vi "pH电极校准.vi"() -> ()   [LabVIEW 2016, in "斯坦道多参数.lvlib"]
uses:
  <vilib>/Utility/miscctls.llb/LVPointTypeDef.ctl
  <vilib>/Analysis/NI_AALBase.lvlib
panel:
  out "通讯状态":string
  in  "电极状态标志":u16(ring) items=["OK", "第一点校正通过", "第二点校正通过", "校正失败,电极零点超出范围", "校正失败,电极斜率超出范围", "第三点校正通过"]
  in  "三点标液3":u16(ring)=6 caption="标液3" items=["TECH4.00", "TECH7.00", "TECH10.00", "NIST1.68", "NIST4.01", "NIST6.86", "NIST9.18", "NIST12.68"]
  in  "三点标液2":u16(ring)=5 caption="标液2" items=["TECH4.00", "TECH7.00", "TECH10.00", "NIST1.68", "NIST4.01", "NIST6.86", "NIST9.18", "NIST12.68"]
  in  "三点标液1":u16(ring)=4 caption="标液1" items=["TECH4.00", "TECH7.00", "TECH10.00", "NIST1.68", "NIST4.01", "NIST6.86", "NIST9.18", "NIST12.68"]
  out "第三点校准值":dbl
  in  "校准停止":bool
  in  "校准启动":bool
  out "第二点校准值":dbl
  out "第一点校准值":dbl
  out "提示":string
  in  "校准模式":enum16{"两点校准", "单点校准", "三点校准"}(ring)
  out "最小值":sgl format="%#.2f"
  out "最大值":sgl format="%#.2f"
  out "变异系数":dbl format="%#.6f"
  out "standard deviation":dbl caption="标准差" format="%#.2f"
  out "mean":dbl caption="均值" format="%#.2f"
  out "波形图表":sgl(graph) caption="历史曲线"
  out "当前检测值":dbl format="%#.2g"
  out "标液2":dbl
  out "标液1":dbl
  out "当前信号值":dbl format="%#.2g"
  out "偏移值补偿":dbl format="%#.2g"
  out "电极斜率":dbl
  out "电极零点":dbl
  # "酸碱度电极设定"
  # "mV"
  # "mV"
  # "%"
  # "pH"
  # "请选择校准模式:"
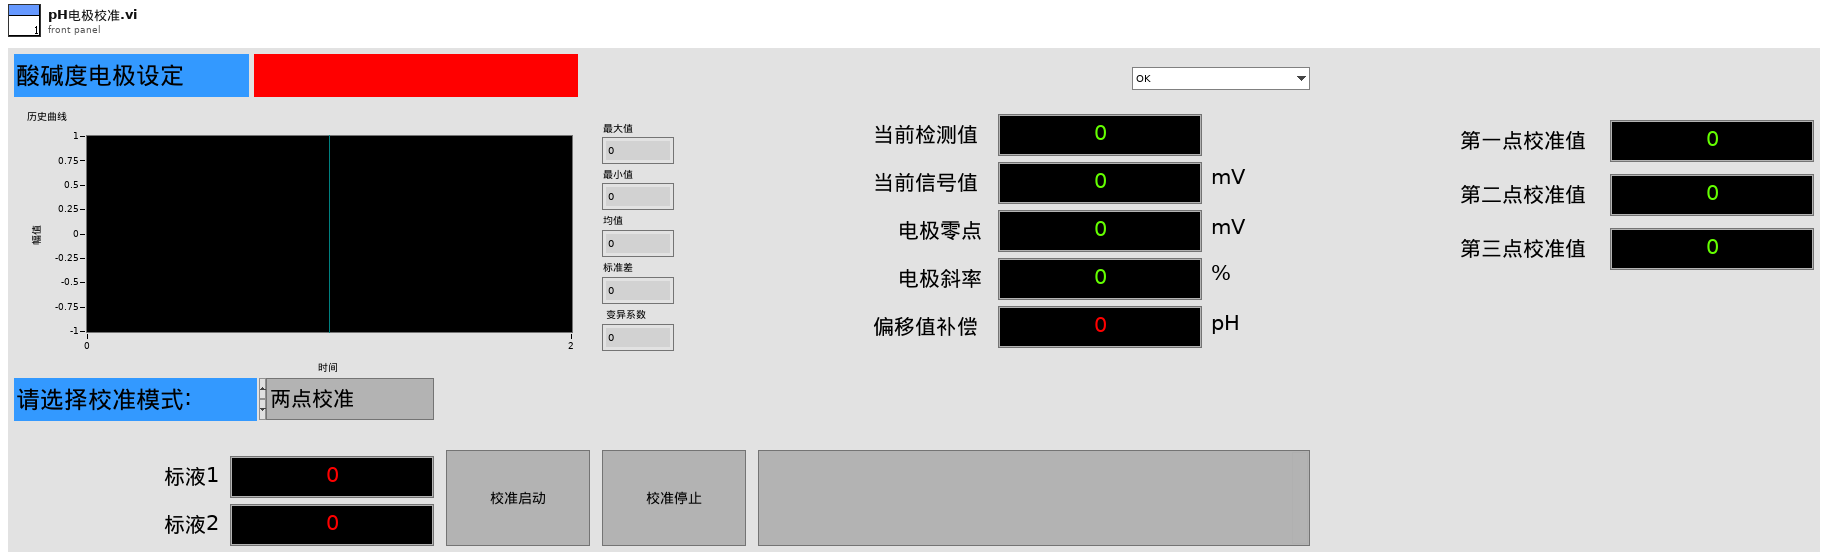
[diagram p1: front panel]
types:
  T1 = typedef "LVPointTypeDef.ctl" = cluster{"Horizontal":i16, "Vertical":i16}
  T2 = typedef "斯坦道多参数.lvlib/校准步骤.ctl" = enum16{"待机", "放置第一点标液", "第一点校准启动", "第一点校准写入", "第一点校准失败", "放置第二点标液", "第二点校准启动", "第二点校准写入", "第二点校准失败", "放置第三点标液", "第三点校准启动", "第三点校准写入", "第三点校准失败", "校准结果写入", "校准结束"}
  T3 = cluster{"电极状态标志":u16, "电极型号标志":u16, "酸碱度测量值":sgl, "温度测量值":sgl, "酸碱度信号值":sgl, "温度信号值":sgl, "酸碱度偏移修正值":sgl, "温度偏移修正值":sgl, "手动温度补偿值":sgl, "酸碱度电极零点":sgl, "酸碱度电极斜率":sgl, "第1点标准值记录":sgl, "第1点信号值记录":sgl, "第1点温度值记录":sgl, "第2点标准值记录":sgl, "第2点信号值记录":sgl, "第2点温度值记录":sgl, "命令滤波设定":u16, "温度模式":enum16{"ATC", "MTC"}, "生产批次":u16, "电极序号":u16, "串口地址":u16, "串口波特率":enum16{"9600", "19200", "115200"}, "串口校验位":enum16{"NONE", "ODD", "EVEN"}, "串口停止位":enum16{"1bit", "2bit"}, "第一点标准值":sgl, "第二点标准值":sgl}
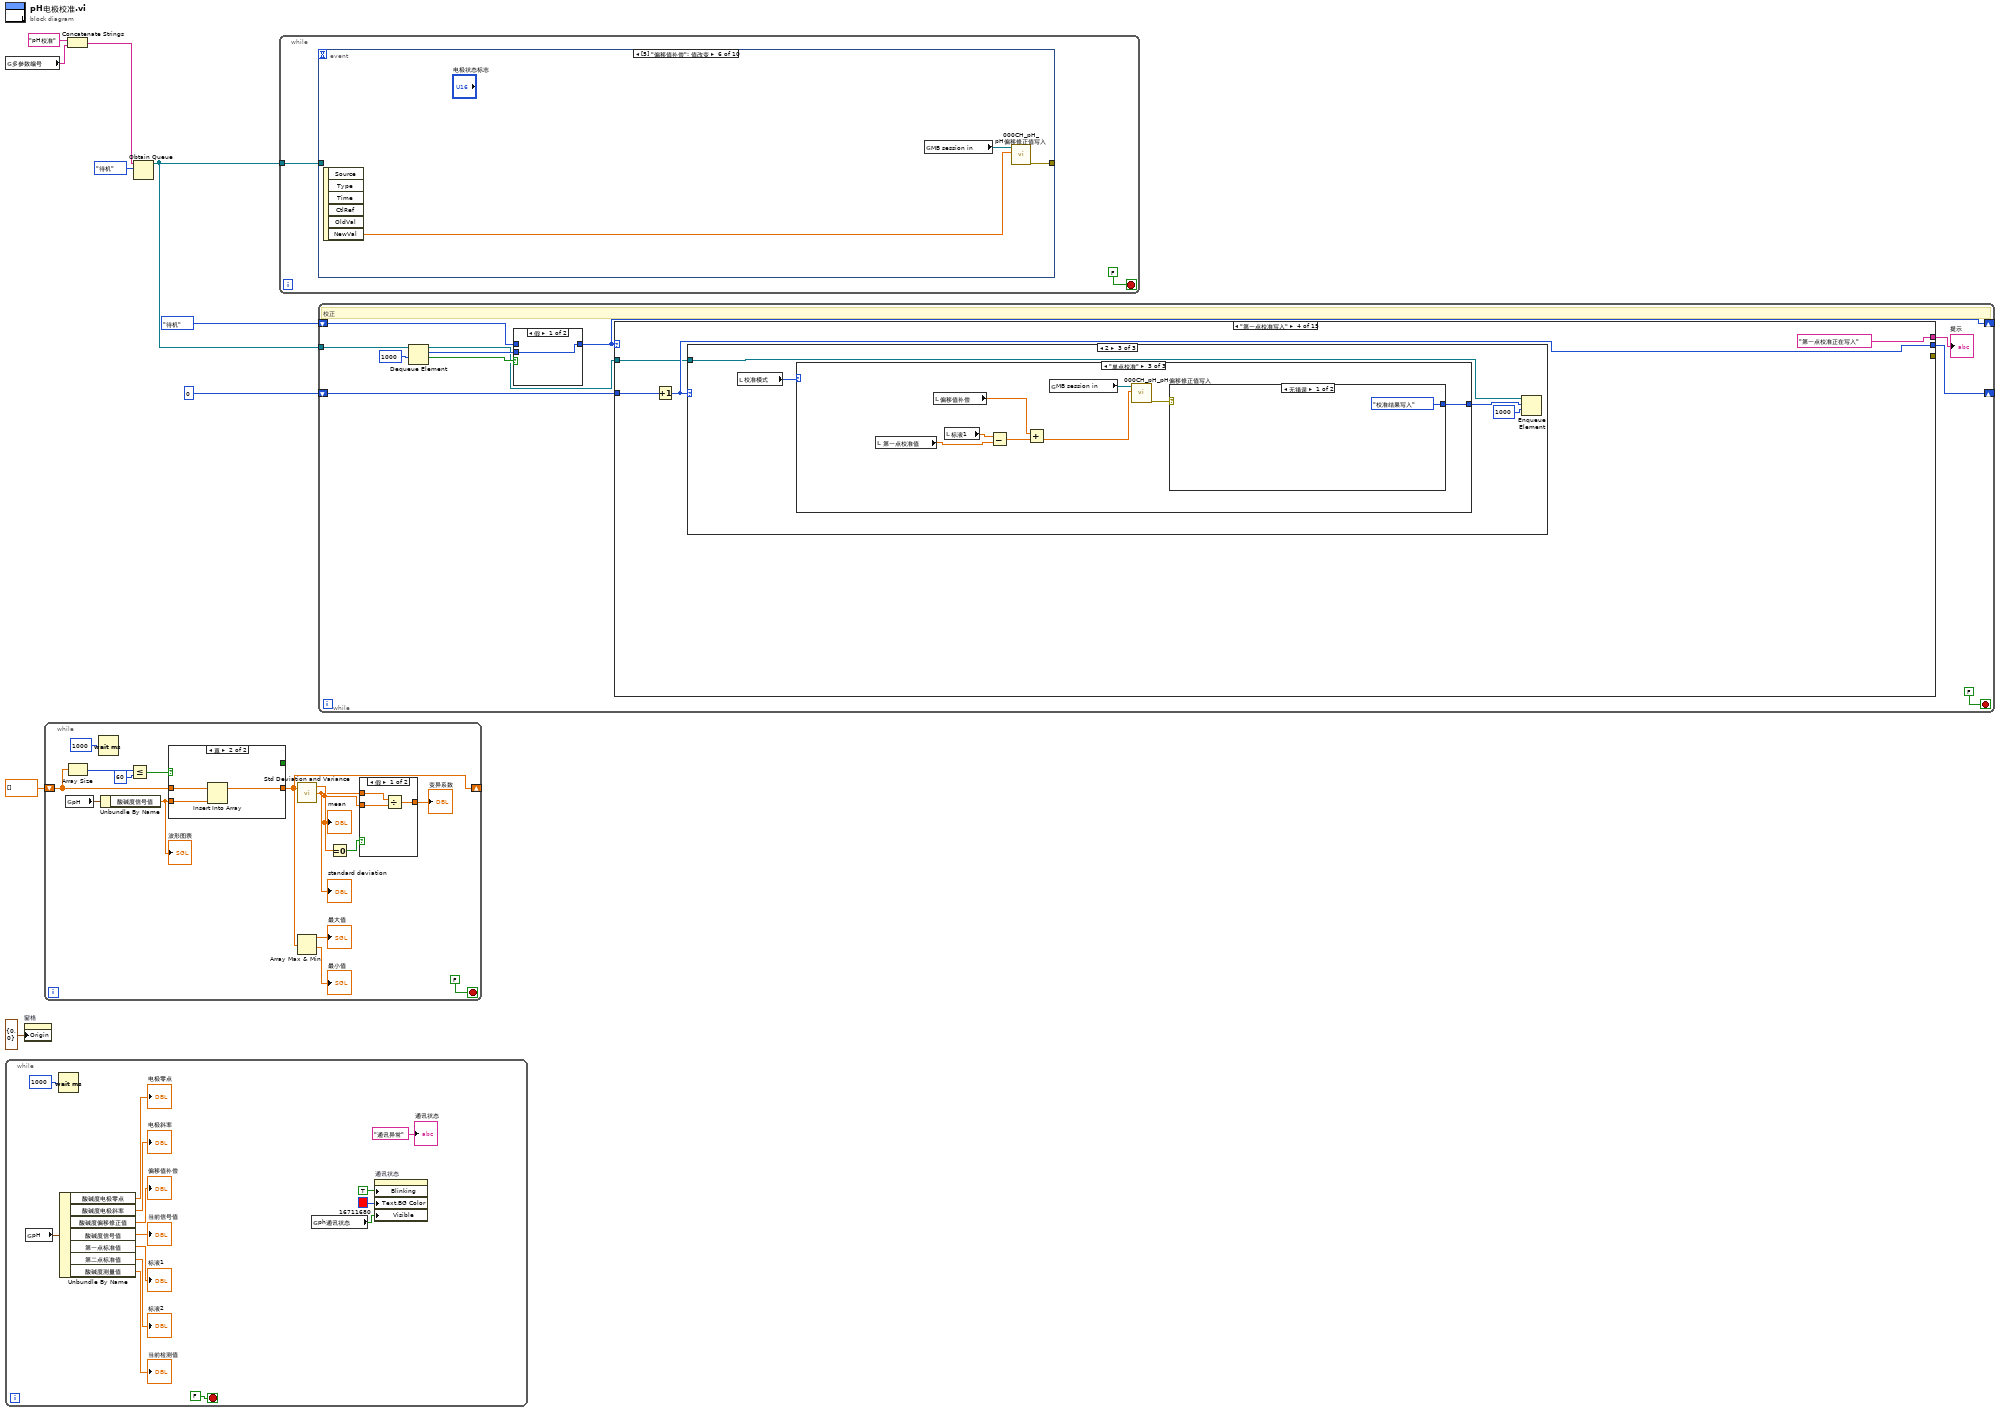
[diagram p0: block diagram]
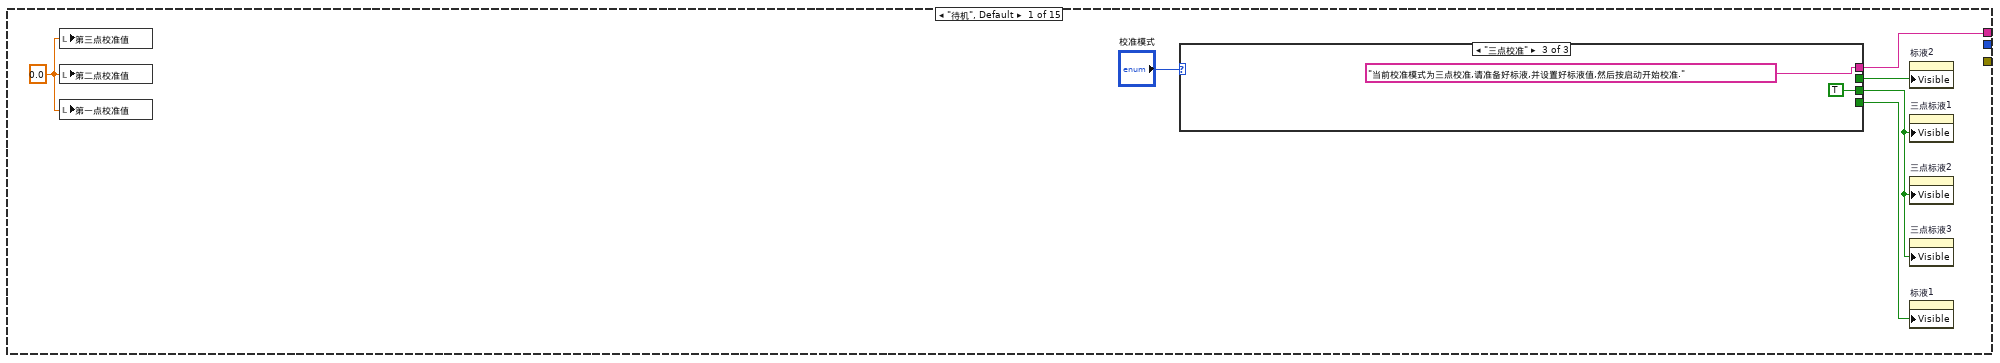
[diagram p3: hidden frame]
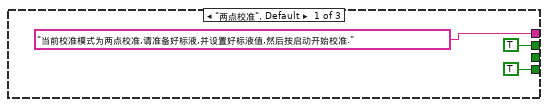
[diagram p4: hidden frame]
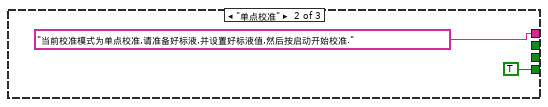
[diagram p5: hidden frame]
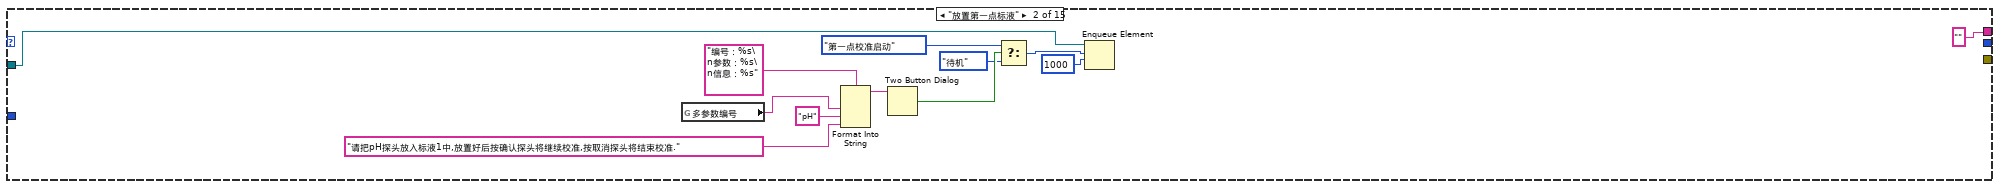
[diagram p6: hidden frame]
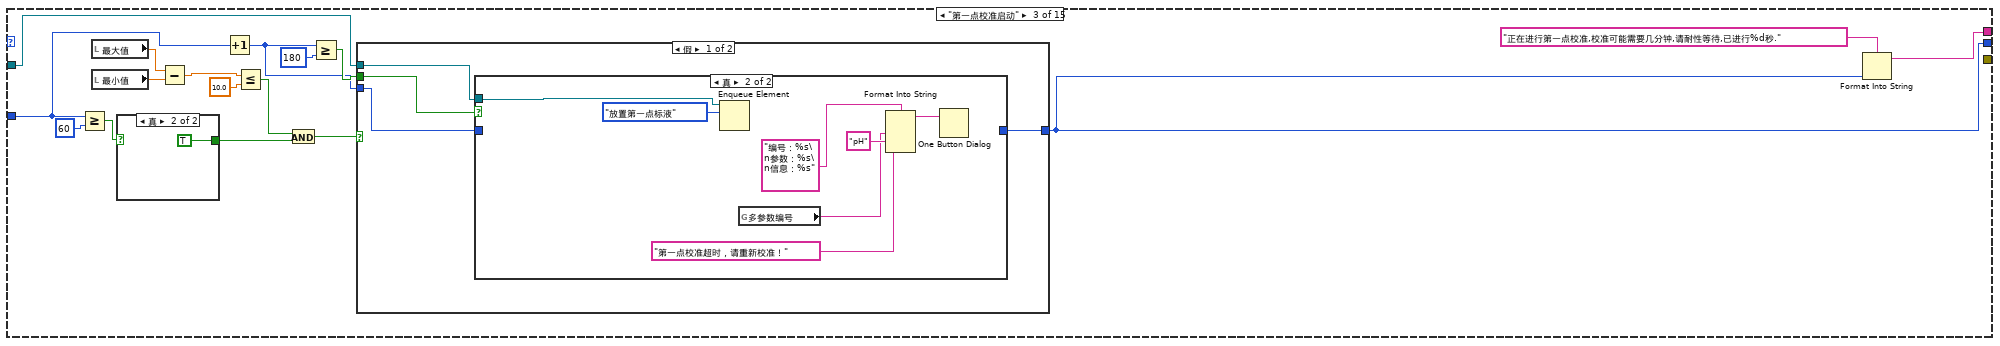
[diagram p7: hidden frame]
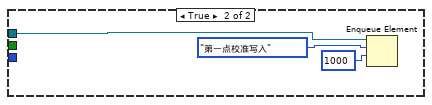
[diagram p9: hidden frame]
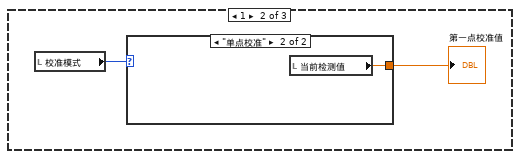
[diagram p12: hidden frame]
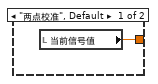
[diagram p13: hidden frame]
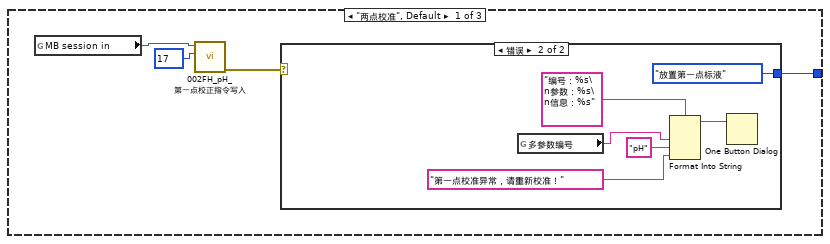
[diagram p14: hidden frame]
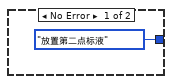
[diagram p15: hidden frame]
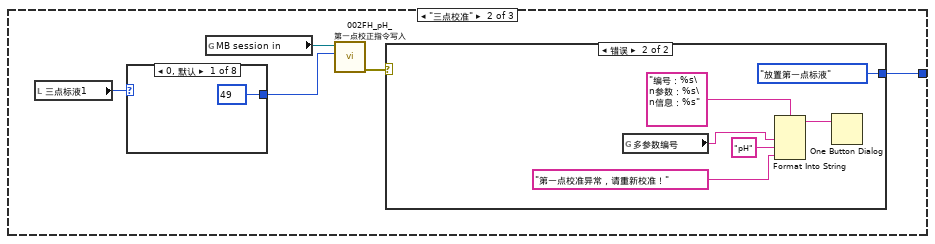
[diagram p16: hidden frame]
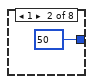
[diagram p17: hidden frame]
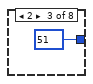
[diagram p18: hidden frame]
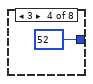
[diagram p19: hidden frame]
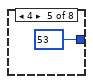
[diagram p20: hidden frame]
diagram:
  n1 = global read "多参数全局变量.vi" "多参数编号"() -> (w1:string)
  n2 = while {
    stop <- FALSE stop-if-true
    n3 = global read "国弘过程全局变量.vi" "pH"() -> (w21:T3)
    n4 = Wait (ms)(milliseconds to wait=u32 1000 ("等待时间（毫秒）")) -> ()  [unwired: 1 out]
    n5 = Unbundle By Name(w21) -> ("酸碱度电极零点"=→"电极零点":sgl, "酸碱度电极斜率"=→"电极斜率":sgl, "酸碱度偏移修正值"=→"偏移值补偿":sgl, "酸碱度信号值"=→"当前信号值":sgl, "第一点标准值"=→"标液1":sgl, "第二点标准值"=→"标液2":sgl, "酸碱度测量值"=→"当前检测值":sgl)
    n6 = global read "多参数全局变量.vi" "ph通讯状态"() -> (w10:bool)
    n7 = property on="通讯状态" class="Str"("Blinking"=TRUE ("闪烁"), "Text.BG Color"=u32 16711680, "Visible"=w10) -> ()  [unwired: 2 in, 2 out]
    "通讯状态" <- "通讯异常" ("当前串口")
  }
  n8 = property on="窗格" class="Pane"("Origin"=T1 {"Horizontal"=0, "Vertical"=0} ("原点")) -> ()  [unwired: 2 in, 2 out]
  n9 = while {
    shift-right: [w30] -> _
    shift-left: sgl[] [] -> [w34]
    stop <- FALSE stop-if-true
    n10 = global read "国弘过程全局变量.vi" "pH"() -> (w31:T3)
    n11 = Array Size(array=w34) -> (size(s)=w36:i32)
    n12 = Wait (ms)(milliseconds to wait=u32 1000 ("等待时间（毫秒）")) -> ()  [unwired: 1 out]
    n13 = Unbundle By Name(w31) -> ("酸碱度信号值"=w24:sgl)
    "波形图表" <- w24
    n14 = Less Or Equal?(x=w36, y=60) -> (x <= y?=w35:bool)
    n15 = case shown="真" w35 {
      tunnel: w34 -> [w47 w50]
      tunnel: w24 -> [w45 w49]
      tunnel: [w43 w48] -> w30
      tunnel: [TRUE _] -> _
      frame False {
        n16 = Replace Array Subset(array=w47, new element=w45) -> (w46:sgl[])  [unwired: 1 in]
        n17 = Rotate 1D Array(1:w46, 2:-1 ("n")) -> (0:w43:sgl[])
      }
      frame True {
        n18 = Insert Into Array(array=w50, new element=w49) -> (w48:sgl[])  [unwired: 1 in]
      }
    }
    n19 = call <vilib>:"Std Deviation and Variance.vi"("X"=w30) -> ("mean"=w26:dbl, "standard deviation"=w25:dbl)  [unwired: 1 in, 1 out]
    "mean" <- w26
    "standard deviation" <- w25
    n20 = Array Max & Min(array=w30) -> (max value=→"最大值":sgl, min value=→"最小值":sgl)  [unwired: 2 out]
    n21 = Equal To 0?(x=w26) -> (x = 0?=w33:bool)
    n22 = case shown="假" w33 {
      tunnel: w25 -> [w41 _]
      tunnel: [w40 _] -> w27
      tunnel: w26 -> [w39 _]
      frame False {
        n23 = Divide(x=w41, y=w39) -> (x/y=w40:dbl)
      }
      frame True {
      }
    }
    "变异系数" <- w27
  }
  n24 = Concatenate Strings("pH校准" ("名称（未命名）"), w1) -> (w2:string)
  n25 = Obtain Queue(name (unnamed)=w2, element data type=校准步骤."待机" ("枚举")) -> (queue out=w4:refnum<queue>)  [unwired: 3 in, 2 out]
  n26 = while {
    tunnel: w4 -> [w51]
    stop <- FALSE stop-if-true
    n27 = event shown="[5] \"偏移值补偿\": 值改变" {
      selector: _ -> [_ _ _ _ _ _ _ _ _ _]
      dyn-events: _ -> [_ _ _ _ _ _ _ _ _ _]
      timeout: _ -> [_ _ _ _ _ _ _ _ _ _]
      tunnel: [_ _ _ _ _ w103 w106 w109 _ _] -> _
      tunnel: w51 -> [_ _ _ _ _ _ _ _ w111 w113]
      event Timeout {
        n28 = event-data() -> ()  [unwired: 1 in, 3 out]
      }
      event "三点标液1": Value Change {
        n29 = event-data() -> ("NewVal"=w53:u16)  [unwired: 1 in, 5 out]
        n30 = case shown="0, 默认" w53 {
          frame 0, Default {
            w54 = u16 0 items=["TECH4.00", "TECH7.00", "TECH10.00", "NIST1.68", "NIST4.01", "NIST6.86", "NIST9.18", "NIST12.68"] ("标液2")
            w55 = u16 2 items=["TECH4.00", "TECH7.00", "TECH10.00", "NIST1.68", "NIST4.01", "NIST6.86", "NIST9.18", "NIST12.68"] ("标液3")
            w56 = u16 1 items=["TECH4.00", "TECH7.00", "TECH10.00", "NIST1.68", "NIST4.01", "NIST6.86", "NIST9.18", "NIST12.68"] ("标液2")
            n31 = local write "三点标液3"(w55) -> ()
            n32 = local write "三点标液2"(w56) -> ()
            n33 = local write "三点标液1"(w54) -> ()
          }
          frame 1 {
            w57 = u16 0 items=["TECH4.00", "TECH7.00", "TECH10.00", "NIST1.68", "NIST4.01", "NIST6.86", "NIST9.18", "NIST12.68"] ("标液2")
            w58 = u16 2 items=["TECH4.00", "TECH7.00", "TECH10.00", "NIST1.68", "NIST4.01", "NIST6.86", "NIST9.18", "NIST12.68"] ("标液3")
            w59 = u16 1 items=["TECH4.00", "TECH7.00", "TECH10.00", "NIST1.68", "NIST4.01", "NIST6.86", "NIST9.18", "NIST12.68"] ("标液2")
            n34 = local write "三点标液3"(w58) -> ()
            n35 = local write "三点标液2"(w59) -> ()
            n36 = local write "三点标液1"(w57) -> ()
          }
          frame 2 {
            w60 = u16 2 items=["TECH4.00", "TECH7.00", "TECH10.00", "NIST1.68", "NIST4.01", "NIST6.86", "NIST9.18", "NIST12.68"] ("标液2")
            w61 = u16 0 items=["TECH4.00", "TECH7.00", "TECH10.00", "NIST1.68", "NIST4.01", "NIST6.86", "NIST9.18", "NIST12.68"] ("标液3")
            w62 = u16 1 items=["TECH4.00", "TECH7.00", "TECH10.00", "NIST1.68", "NIST4.01", "NIST6.86", "NIST9.18", "NIST12.68"] ("标液2")
            n37 = local write "三点标液3"(w61) -> ()
            n38 = local write "三点标液2"(w62) -> ()
            n39 = local write "三点标液1"(w60) -> ()
          }
          frame 3 {
            w63 = u16 3 items=["TECH4.00", "TECH7.00", "TECH10.00", "NIST1.68", "NIST4.01", "NIST6.86", "NIST9.18", "NIST12.68"] ("标液2")
            w64 = u16 5 items=["TECH4.00", "TECH7.00", "TECH10.00", "NIST1.68", "NIST4.01", "NIST6.86", "NIST9.18", "NIST12.68"] ("标液3")
            w65 = u16 4 items=["TECH4.00", "TECH7.00", "TECH10.00", "NIST1.68", "NIST4.01", "NIST6.86", "NIST9.18", "NIST12.68"] ("标液2")
            n40 = local write "三点标液3"(w64) -> ()
            n41 = local write "三点标液2"(w65) -> ()
            n42 = local write "三点标液1"(w63) -> ()
          }
          frame 4 {
            w66 = u16 4 items=["TECH4.00", "TECH7.00", "TECH10.00", "NIST1.68", "NIST4.01", "NIST6.86", "NIST9.18", "NIST12.68"] ("标液2")
            w67 = u16 6 items=["TECH4.00", "TECH7.00", "TECH10.00", "NIST1.68", "NIST4.01", "NIST6.86", "NIST9.18", "NIST12.68"] ("标液3")
            w68 = u16 5 items=["TECH4.00", "TECH7.00", "TECH10.00", "NIST1.68", "NIST4.01", "NIST6.86", "NIST9.18", "NIST12.68"] ("标液2")
            n43 = local write "三点标液3"(w67) -> ()
            n44 = local write "三点标液2"(w68) -> ()
            n45 = local write "三点标液1"(w66) -> ()
          }
          frame 5..7 {
            w69 = u16 5 items=["TECH4.00", "TECH7.00", "TECH10.00", "NIST1.68", "NIST4.01", "NIST6.86", "NIST9.18", "NIST12.68"] ("标液2")
            w70 = u16 7 items=["TECH4.00", "TECH7.00", "TECH10.00", "NIST1.68", "NIST4.01", "NIST6.86", "NIST9.18", "NIST12.68"] ("标液3")
            w71 = u16 6 items=["TECH4.00", "TECH7.00", "TECH10.00", "NIST1.68", "NIST4.01", "NIST6.86", "NIST9.18", "NIST12.68"] ("标液2")
            n46 = local write "三点标液3"(w70) -> ()
            n47 = local write "三点标液2"(w71) -> ()
            n48 = local write "三点标液1"(w69) -> ()
          }
        }
      }
      event "三点标液2": Value Change {
        n49 = event-data() -> ("NewVal"=w72:u16)  [unwired: 1 in, 5 out]
        n50 = case shown="6, 7" w72 {
          frame 0..2, Default {
            w73 = u16 0 items=["TECH4.00", "TECH7.00", "TECH10.00", "NIST1.68", "NIST4.01", "NIST6.86", "NIST9.18", "NIST12.68"] ("标液2")
            w74 = u16 2 items=["TECH4.00", "TECH7.00", "TECH10.00", "NIST1.68", "NIST4.01", "NIST6.86", "NIST9.18", "NIST12.68"] ("标液3")
            w75 = u16 1 items=["TECH4.00", "TECH7.00", "TECH10.00", "NIST1.68", "NIST4.01", "NIST6.86", "NIST9.18", "NIST12.68"] ("标液2")
            n51 = local write "三点标液3"(w74) -> ()
            n52 = local write "三点标液2"(w75) -> ()
            n53 = local write "三点标液1"(w73) -> ()
          }
          frame 3, 4 {
            w76 = u16 3 items=["TECH4.00", "TECH7.00", "TECH10.00", "NIST1.68", "NIST4.01", "NIST6.86", "NIST9.18", "NIST12.68"] ("标液2")
            w77 = u16 5 items=["TECH4.00", "TECH7.00", "TECH10.00", "NIST1.68", "NIST4.01", "NIST6.86", "NIST9.18", "NIST12.68"] ("标液3")
            w78 = u16 4 items=["TECH4.00", "TECH7.00", "TECH10.00", "NIST1.68", "NIST4.01", "NIST6.86", "NIST9.18", "NIST12.68"] ("标液2")
            n54 = local write "三点标液3"(w77) -> ()
            n55 = local write "三点标液2"(w78) -> ()
            n56 = local write "三点标液1"(w76) -> ()
          }
          frame 5 {
            w79 = u16 6 items=["TECH4.00", "TECH7.00", "TECH10.00", "NIST1.68", "NIST4.01", "NIST6.86", "NIST9.18", "NIST12.68"] ("标液3")
            w80 = u16 5 items=["TECH4.00", "TECH7.00", "TECH10.00", "NIST1.68", "NIST4.01", "NIST6.86", "NIST9.18", "NIST12.68"] ("标液2")
            n57 = local write "三点标液3"(w79) -> ()
            n58 = local write "三点标液2"(w80) -> ()
          }
          frame 6, 7 {
            w81 = u16 7 items=["TECH4.00", "TECH7.00", "TECH10.00", "NIST1.68", "NIST4.01", "NIST6.86", "NIST9.18", "NIST12.68"] ("标液3")
            w82 = u16 6 items=["TECH4.00", "TECH7.00", "TECH10.00", "NIST1.68", "NIST4.01", "NIST6.86", "NIST9.18", "NIST12.68"] ("标液2")
            n59 = local write "三点标液3"(w81) -> ()
            n60 = local write "三点标液2"(w82) -> ()
          }
        }
      }
      event "三点标液3": Value Change {
        n61 = event-data() -> ("NewVal"=w83:u16)  [unwired: 1 in, 5 out]
        n62 = case shown="3..7" w83 {
          frame 0, 1, Default {
            w84 = u16 2 items=["TECH4.00", "TECH7.00", "TECH10.00", "NIST1.68", "NIST4.01", "NIST6.86", "NIST9.18", "NIST12.68"] ("标液2")
            w85 = u16 0 items=["TECH4.00", "TECH7.00", "TECH10.00", "NIST1.68", "NIST4.01", "NIST6.86", "NIST9.18", "NIST12.68"] ("标液3")
            w86 = u16 1 items=["TECH4.00", "TECH7.00", "TECH10.00", "NIST1.68", "NIST4.01", "NIST6.86", "NIST9.18", "NIST12.68"] ("标液2")
            n63 = local write "三点标液3"(w85) -> ()
            n64 = local write "三点标液2"(w86) -> ()
            n65 = local write "三点标液1"(w84) -> ()
          }
          frame 2 {
            w87 = u16 0 items=["TECH4.00", "TECH7.00", "TECH10.00", "NIST1.68", "NIST4.01", "NIST6.86", "NIST9.18", "NIST12.68"] ("标液2")
            w88 = u16 2 items=["TECH4.00", "TECH7.00", "TECH10.00", "NIST1.68", "NIST4.01", "NIST6.86", "NIST9.18", "NIST12.68"] ("标液3")
            w89 = u16 1 items=["TECH4.00", "TECH7.00", "TECH10.00", "NIST1.68", "NIST4.01", "NIST6.86", "NIST9.18", "NIST12.68"] ("标液2")
            n66 = local write "三点标液3"(w88) -> ()
            n67 = local write "三点标液2"(w89) -> ()
            n68 = local write "三点标液1"(w87) -> ()
          }
          frame 3..7 {
            n69 = local read "三点标液1"() -> (w92:u16)
            n70 = local read "三点标液2"() -> (w91:u16)
            n71 = Less?(x=w92, y=w91) -> (x < y?=w90:bool)
            n72 = case shown="假" w90 {
              frame False {
              }
              frame True {
                n73 = local read "三点标液3"() -> (w95:u16)
                n74 = local read "三点标液2"() -> (w93:u16)
                n75 = Less Or Equal?(x=w95, y=w93) -> (x <= y?=w94:bool)
                n76 = case shown="真" w94 {
                  tunnel: w93 -> [_ w97]
                  frame False {
                  }
                  frame True {
                    n77 = Increment(x=w97) -> (x+1=w96:u16)
                    n78 = local write "三点标液3"(w96) -> ()
                  }
                }
              }
            }
          }
        }
      }
      event "标液1", "标液2", "偏移值补偿": Mouse Down {
        n79 = event-data() -> ("CtlRef"=w101:refnum<vi>)  [unwired: 1 in, 7 out]
        n80 = property class="DigNum (严格)"(reference=w101) -> (reference out=w98:refnum<vi>, "Value"=w99:dbl)  [unwired: 1 in, 1 out]
        n81 = call "数字键盘.vi"("OldNumber"=w99) -> ("NewNumber"=w100:dbl)  [unwired: 1 in]
        n82 = property class="DigNum (严格)"(reference=w98, "Val(Sgnl)"=w100) -> ()  [unwired: 1 in, 2 out]
      }
      event "偏移值补偿": Value Change {
        n83 = event-data() -> ("NewVal"=w104:dbl)  [unwired: 1 in, 5 out]
        n84 = global read "多参数全局变量.vi" "MB session in"() -> (w102:refnum<class "MB_Master.lvclass">)
        n85 = call "000CH_pH_pH偏移修正值写入.vi"("数值"=w104, "MB session in"=w102) -> ("error out"=w103:errorcluster)  [unwired: 8 in, 1 out]
      }
      event "标液1": Value Change {
        n86 = event-data() -> ("NewVal"=w107:dbl)  [unwired: 1 in, 5 out]
        n87 = global read "多参数全局变量.vi" "MB session in"() -> (w105:refnum<class "MB_Master.lvclass">)
        n88 = call "0030H_pH_第一点标准值写入.vi"("数值"=w107, "MB session in"=w105) -> ("error out"=w106:errorcluster)  [unwired: 8 in, 1 out]
      }
      event "标液2": Value Change {
        n89 = event-data() -> ("NewVal"=w110:dbl)  [unwired: 1 in, 5 out]
        n90 = global read "多参数全局变量.vi" "MB session in"() -> (w108:refnum<class "MB_Master.lvclass">)
        n91 = call "0033H_pH_第二点标准值写入.vi"("数值"=w110, "MB session in"=w108) -> ("error out"=w109:errorcluster)  [unwired: 8 in, 1 out]
      }
      event "校准启动": Value Change {
        n92 = event-data() -> ()  [unwired: 1 in, 6 out]
        n93 = Enqueue Element(queue=w111, element=校准步骤."放置第一点标液" ("元素")) -> ()  [unwired: 2 in, 3 out]
      }
      event "校准停止": Value Change {
        n94 = event-data() -> ()  [unwired: 1 in, 6 out]
        n95 = Flush Queue(queue=w113) -> (queue out=w114:refnum<queue>)  [unwired: 1 in, 2 out]
        n96 = Enqueue Element(queue=w114, element=校准步骤."待机" ("元素"), timeout in ms (-1)=1000 ("超时毫秒(-1)")) -> ()  [unwired: 1 in, 3 out]
      }
    }
  }
  n97 = while "While循环" {
    shift-right: [w118] -> _
    shift-left: 校准步骤."待机" ("枚举") -> [w119]
    shift-right: [w125] -> _
    shift-left: 0 -> [w126]
    tunnel: w4 -> [w123]
    stop <- FALSE stop-if-true
    # "校正"
    n98 = Dequeue Element(queue=w123, timeout in ms (-1)=1000 ("超时毫秒(-1)")) -> (queue out=w117:refnum<queue>, element=w120:T2, timed out?=w121:bool)  [unwired: 1 in, 1 out]
    n99 = case shown="假" w121 {
      tunnel: w120 -> [w128 _]
      tunnel: [w128 w129] -> w118
      tunnel: w119 -> [_ w129]
      frame False {
      }
      frame True {
      }
    }
    n100 = case shown="\"第一点校准写入\"" w118 {
      tunnel: [w135 "" ("提示") w170 "第一点校准正在写入" ("提示") _ "" ("提示") w273 "第二点校准正在写入" ("提示") _ "" ("提示") w358 "第三点校准正在写入" ("提示") _ w406 w444] -> w124
      tunnel: w126 -> [_ _ w164 w190 _ _ w267 w293 _ _ w352 w378 _ _ _]
      tunnel: [_ _ w155 w189 _ _ w258 w292 _ _ w343 w377 _ _ _] -> w125
      tunnel: w117 -> [_ w154 w158 w188 _ w257 w261 w291 _ w342 w346 w376 _ w413 _]
      tunnel: [_ _ _ _ _ _ _ _ _ _ _ _ _ w410 _] -> _
      frame "待机", Default {
        w131 = 0.0 ("第一点校准值")
        n101 = local write "第三点校准值"(w131) -> ()
        n102 = local write "第二点校准值"(w131) -> ()
        n103 = local write "第一点校准值"(w131) -> ()
        n104 = case shown="\"三点校准\"" "校准模式" {
          tunnel: ["当前校准模式为两点校准,请准备好标液,并设置好标液值,然后按启动开始校准." ("提示") "当前校准模式为单点校准,请准备好标液,并设置好标液值,然后按启动开始校准." ("提示") "当前校准模式为三点校准,请准备好标液,并设置好标液值,然后按启动开始校准." ("提示")] -> w135
          tunnel: [TRUE ("可见") _ _] -> w134
          tunnel: [TRUE ("可见") TRUE ("可见") _] -> w132
          tunnel: [_ _ TRUE ("可见")] -> w130
          frame "两点校准", Default {
          }
          frame "单点校准" {
          }
          frame "三点校准" {
          }
        }
        n105 = property on="标液2" class="DigNum (严格)"("Visible"=w134) -> ()  [unwired: 2 in, 2 out]
        n106 = property on="三点标液1" class="Ring (严格)"("Visible"=w130) -> ()  [unwired: 2 in, 2 out]
        n107 = property on="三点标液2" class="Ring (严格)"("Visible"=w130) -> ()  [unwired: 2 in, 2 out]
        n108 = property on="三点标液3" class="Ring (严格)"("Visible"=w130) -> ()  [unwired: 2 in, 2 out]
        n109 = property on="标液1" class="DigNum (严格)"("Visible"=w132) -> ()  [unwired: 2 in, 2 out]
      }
      frame "放置第一点标液" {
        n110 = global read "多参数全局变量.vi" "多参数编号"() -> (w146:string)
        n111 = Format Into String(format string="编号：%s\n参数：%s\n信息：%s" ("格式字符串"), w146, "pH" ("输入 2"), "请把pH探头放入标液1中,放置好后按确认探头将继续校准,按取消探头将结束校准." ("消息")) -> (resulting string=w143:string)  [unwired: 2 in, 1 out]
        n112 = Two Button Dialog(message=w143) -> (T button?=w152:bool)  [unwired: 2 in]
        n113 = Select(t=校准步骤."第一点校准启动" ("元素"), s=w152, f=校准步骤."待机" ("元素")) -> (s? t:f=w149:T2)
        n114 = Enqueue Element(queue=w154, element=w149, timeout in ms (-1)=1000 ("超时毫秒(-1)")) -> ()  [unwired: 1 in, 3 out]
      }
      frame "第一点校准启动" {
        n115 = Greater Or Equal?(x=w164, y=60) -> (x >= y?=w165:bool)
        n116 = local read "最大值"() -> (w161:sgl)
        n117 = local read "最小值"() -> (w162:sgl)
        n118 = case shown="真" w165 {
          tunnel: [_ TRUE] -> w163
          frame False {
          }
          frame True {
          }
        }
        n119 = Subtract(x=w161, y=w162) -> (x-y=w160:sgl)
        n120 = Increment(x=w164) -> (x+1=w156:i32)
        n121 = Less Or Equal?(x=w160, y=10.0) -> (x <= y?=w168:bool)
        n122 = And(x=w168, y=w163) -> (x .and. y?=w159:bool)
        n123 = Greater Or Equal?(x=w156, y=180) -> (x >= y?=w157:bool)
        n124 = case shown="假" w159 {
          tunnel: w158 -> [w174 w186]
          tunnel: w157 -> [w175 _]
          tunnel: w156 -> [w173 _]
          tunnel: [w172 _] -> w155
          frame False {
            n125 = case shown="真" w175 {
              tunnel: w174 -> [_ w183]
              tunnel: w173 -> [w176 _]
              tunnel: [w176 _] -> w172
              frame False {
              }
              frame True {
                n126 = Enqueue Element(queue=w183, element=校准步骤."放置第一点标液" ("元素")) -> ()  [unwired: 2 in, 3 out]
                n127 = global read "多参数全局变量.vi" "多参数编号"() -> (w178:string)
                n128 = Format Into String(format string="编号：%s\n参数：%s\n信息：%s" ("格式字符串"), w178, "pH" ("输入 2"), "第一点校准超时，请重新校准！" ("error source (\" \")")) -> (resulting string=w180:string)  [unwired: 2 in, 1 out]
                n129 = One Button Dialog(message=w180) -> ()  [unwired: 1 in, 1 out]
              }
            }
          }
          frame True {
            n130 = Enqueue Element(queue=w186, element=校准步骤."第一点校准写入" ("元素"), timeout in ms (-1)=1000 ("超时毫秒(-1)")) -> ()  [unwired: 1 in, 3 out]
          }
        }
        n131 = Format Into String(format string="正在进行第一点校准,校准可能需要几分钟,请耐性等待,已进行%d秒." ("格式字符串"), w155) -> (resulting string=w170:string)  [unwired: 2 in, 1 out]
      }
      frame "第一点校准写入" {
        n132 = Increment(x=w190) -> (x+1=w189:i32)
        n133 = case shown="2" w189 {
          tunnel: w188 -> [_ _ w199]
          frame 0, Default {
          }
          frame 1 {
            n134 = local read "校准模式"() -> (w192:enum16{"两点校准", "单点校准", "三点校准"})
            n135 = case shown="\"单点校准\"" w192 {
              tunnel: [w194 w195] -> w193
              frame "两点校准", Default {
                n136 = local read "当前信号值"() -> (w194:dbl)
              }
              frame "单点校准" {
                n137 = local read "当前检测值"() -> (w195:dbl)
              }
            }
            "第一点校准值" <- w193
          }
          frame 2 {
            n138 = local read "校准模式"() -> (w198:enum16{"两点校准", "单点校准", "三点校准"})
            n139 = case shown="\"单点校准\"" w198 {
              tunnel: [w203 w215 w233] -> w197
              frame "两点校准", Default {
                n140 = global read "多参数全局变量.vi" "MB session in"() -> (w202:refnum<class "MB_Master.lvclass">)
                n141 = call "002FH_pH_第一点校正指令写入.vi"("数值"=u16 17, "MB session in"=w202) -> ("error out"=w200:errorcluster)  [unwired: 8 in, 1 out]
                n142 = case shown="错误" w200 {
                  tunnel: [校准步骤."放置第二点标液" ("元素") 校准步骤."放置第一点标液" ("元素")] -> w203
                  frame No Error {
                  }
                  frame Error {
                    n143 = global read "多参数全局变量.vi" "多参数编号"() -> (w206:string)
                    n144 = Format Into String(format string="编号：%s\n参数：%s\n信息：%s" ("格式字符串"), w206, "pH" ("输入 2"), "第一点校准异常，请重新校准！" ("error source (\" \")")) -> (resulting string=w208:string)  [unwired: 2 in, 1 out]
                    n145 = One Button Dialog(message=w208) -> ()  [unwired: 1 in, 1 out]
                  }
                }
              }
              frame "三点校准" {
                n146 = local read "三点标液1"() -> (w212:u16)
                n147 = case shown="0, 默认" w212 {
                  tunnel: [u16 49 ("数值") u16 50 ("数值") u16 51 ("数值") u16 52 ("数值") u16 53 ("数值") u16 54 ("数值") u16 55 ("数值") u16 56 ("数值")] -> w211
                  frame 0, Default {
                  }
                  frame 1 {
                  }
                  frame 2 {
                  }
                  frame 3 {
                  }
                  frame 4 {
                  }
                  frame 5 {
                  }
                  frame 6 {
                  }
                  frame 7 {
                  }
                }
                n148 = global read "多参数全局变量.vi" "MB session in"() -> (w214:refnum<class "MB_Master.lvclass">)
                n149 = call "002FH_pH_第一点校正指令写入.vi"("数值"=w211, "MB session in"=w214) -> ("error out"=w213:errorcluster)  [unwired: 8 in, 1 out]
                n150 = case shown="错误" w213 {
                  tunnel: [校准步骤."放置第二点标液" ("元素") 校准步骤."放置第一点标液" ("元素")] -> w215
                  frame No Error {
                  }
                  frame Error {
                    n151 = global read "多参数全局变量.vi" "多参数编号"() -> (w226:string)
                    n152 = Format Into String(format string="编号：%s\n参数：%s\n信息：%s" ("格式字符串"), w226, "pH" ("输入 2"), "第一点校准异常，请重新校准！" ("error source (\" \")")) -> (resulting string=w228:string)  [unwired: 2 in, 1 out]
                    n153 = One Button Dialog(message=w228) -> ()  [unwired: 1 in, 1 out]
                  }
                }
              }
              frame "单点校准" {
                n154 = local read "第一点校准值"() -> (w238:dbl)
                n155 = local read "偏移值补偿"() -> (w231:dbl)
                n156 = local read "标液1"() -> (w237:dbl)
                n157 = Subtract(x=w237, y=w238) -> (x-y=w235:dbl)
                n158 = Add(x=w231, y=w235) -> (x+y=w232:dbl)
                n159 = global read "多参数全局变量.vi" "MB session in"() -> (w236:refnum<class "MB_Master.lvclass">)
                n160 = call "000CH_pH_pH偏移修正值写入.vi"("数值"=w232, "MB session in"=w236) -> ("error out"=w234:errorcluster)  [unwired: 8 in, 1 out]
                n161 = case shown="无错误" w234 {
                  tunnel: [校准步骤."校准结果写入" ("元素") 校准步骤."放置第一点标液" ("元素")] -> w233
                  frame No Error {
                  }
                  frame Error {
                    n162 = global read "多参数全局变量.vi" "多参数编号"() -> (w243:string)
                    n163 = Format Into String(format string="编号：%s\n参数：%s\n信息：%s" ("格式字符串"), w243, "pH" ("输入 2"), "校准异常，请重新校准！" ("error source (\" \")")) -> (resulting string=w241:string)  [unwired: 2 in, 1 out]
                    n164 = One Button Dialog(message=w241) -> ()  [unwired: 1 in, 1 out]
                  }
                }
              }
            }
            n165 = Enqueue Element(queue=w199, element=w197, timeout in ms (-1)=1000 ("超时毫秒(-1)")) -> ()  [unwired: 1 in, 3 out]
          }
        }
      }
      frame "第一点校准失败" {
      }
      frame "放置第二点标液" {
        n166 = global read "多参数全局变量.vi" "多参数编号"() -> (w249:string)
        n167 = Format Into String(format string="编号：%s\n参数：%s\n信息：%s" ("格式字符串"), w249, "pH" ("输入 2"), "请把探头放入标液2中,放置好后按确认探头将继续校准,按取消探头将结束校准." ("消息")) -> (resulting string=w246:string)  [unwired: 2 in, 1 out]
        n168 = Two Button Dialog(message=w246) -> (T button?=w255:bool)  [unwired: 2 in]
        n169 = Select(t=校准步骤."第二点校准启动" ("元素"), s=w255, f=校准步骤."待机" ("元素")) -> (s? t:f=w252:T2)
        n170 = Enqueue Element(queue=w257, element=w252, timeout in ms (-1)=1000 ("超时毫秒(-1)")) -> ()  [unwired: 1 in, 3 out]
      }
      frame "第二点校准启动" {
        n171 = Greater Or Equal?(x=w267, y=60) -> (x >= y?=w268:bool)
        n172 = local read "最大值"() -> (w264:sgl)
        n173 = local read "最小值"() -> (w265:sgl)
        n174 = case shown="真" w268 {
          tunnel: [_ TRUE] -> w266
          frame False {
          }
          frame True {
          }
        }
        n175 = Subtract(x=w264, y=w265) -> (x-y=w263:sgl)
        n176 = Increment(x=w267) -> (x+1=w259:i32)
        n177 = Less Or Equal?(x=w263, y=10.0) -> (x <= y?=w271:bool)
        n178 = And(x=w271, y=w266) -> (x .and. y?=w262:bool)
        n179 = Greater Or Equal?(x=w259, y=180) -> (x >= y?=w260:bool)
        n180 = case shown="假" w262 {
          tunnel: w261 -> [w277 w289]
          tunnel: w260 -> [w278 _]
          tunnel: w259 -> [w276 _]
          tunnel: [w275 _] -> w258
          frame False {
            n181 = case shown="真" w278 {
              tunnel: w277 -> [_ w286]
              tunnel: w276 -> [w279 _]
              tunnel: [w279 _] -> w275
              frame False {
              }
              frame True {
                n182 = Enqueue Element(queue=w286, element=校准步骤."放置第二点标液" ("元素")) -> ()  [unwired: 2 in, 3 out]
                n183 = global read "多参数全局变量.vi" "多参数编号"() -> (w281:string)
                n184 = Format Into String(format string="编号：%s\n参数：%s\n信息：%s" ("格式字符串"), w281, "pH" ("输入 2"), "第二点校准超时，请重新校准！" ("error source (\" \")")) -> (resulting string=w283:string)  [unwired: 2 in, 1 out]
                n185 = One Button Dialog(message=w283) -> ()  [unwired: 1 in, 1 out]
              }
            }
          }
          frame True {
            n186 = Enqueue Element(queue=w289, element=校准步骤."第二点校准写入" ("元素"), timeout in ms (-1)=1000 ("超时毫秒(-1)")) -> ()  [unwired: 1 in, 3 out]
          }
        }
        n187 = Format Into String(format string="正在进行第二点校准,校准可能需要几分钟,请耐性等待,已进行%d秒." ("格式字符串"), w258) -> (resulting string=w273:string)  [unwired: 2 in, 1 out]
      }
      frame "第二点校准写入" {
        n188 = Increment(x=w293) -> (x+1=w292:i32)
        n189 = case shown="1" w292 {
          tunnel: w291 -> [_ _ w299]
          frame 0, Default {
          }
          frame 1 {
            n190 = local read "当前信号值"() -> (→"第二点校准值":dbl)
          }
          frame 2 {
            n191 = local read "校准模式"() -> (w296:enum16{"两点校准", "单点校准", "三点校准"})
            n192 = case shown="\"三点校准\"" w296 {
              tunnel: [w300 w313] -> w297
              frame "两点校准", Default {
                n193 = global read "多参数全局变量.vi" "MB session in"() -> (w302:refnum<class "MB_Master.lvclass">)
                n194 = call "0032H_pH_第二点校正指令写入.vi"("数值"=u16 33, "MB session in"=w302) -> ("error out"=w301:errorcluster)  [unwired: 8 in, 1 out]
                n195 = case shown="错误" w301 {
                  tunnel: [校准步骤."校准结果写入" ("元素") 校准步骤."放置第二点标液" ("元素")] -> w300
                  frame No Error {
                  }
                  frame Error {
                    n196 = global read "多参数全局变量.vi" "多参数编号"() -> (w306:string)
                    n197 = Format Into String(format string="编号：%s\n参数：%s\n信息：%s" ("格式字符串"), w306, "pH" ("输入 2"), "第二点校准异常，请重新校准！" ("error source (\" \")")) -> (resulting string=w308:string)  [unwired: 2 in, 1 out]
                    n198 = One Button Dialog(message=w308) -> ()  [unwired: 1 in, 1 out]
                  }
                }
              }
              frame "三点校准" {
                n199 = local read "三点标液2"() -> (w312:u16)
                n200 = case shown="7" w312 {
                  tunnel: [u16 49 ("数值") u16 50 ("数值") u16 51 ("数值") u16 52 ("数值") u16 53 ("数值") u16 54 ("数值") u16 55 ("数值") u16 56 ("数值")] -> w311
                  frame 0, Default {
                  }
                  frame 1 {
                  }
                  frame 2 {
                  }
                  frame 3 {
                  }
                  frame 4 {
                  }
                  frame 5 {
                  }
                  frame 6 {
                  }
                  frame 7 {
                  }
                }
                n201 = global read "多参数全局变量.vi" "MB session in"() -> (w315:refnum<class "MB_Master.lvclass">)
                n202 = call "0032H_pH_第二点校正指令写入.vi"("数值"=w311, "MB session in"=w315) -> ("error out"=w314:errorcluster)  [unwired: 8 in, 1 out]
                n203 = case shown="错误" w314 {
                  tunnel: [校准步骤."放置第三点标液" ("元素") 校准步骤."放置第二点标液" ("元素")] -> w313
                  frame No Error {
                  }
                  frame Error {
                    n204 = global read "多参数全局变量.vi" "多参数编号"() -> (w326:string)
                    n205 = Format Into String(format string="编号：%s\n参数：%s\n信息：%s" ("格式字符串"), w326, "pH" ("输入 2"), "第二点校准异常，请重新校准！" ("error source (\" \")")) -> (resulting string=w328:string)  [unwired: 2 in, 1 out]
                    n206 = One Button Dialog(message=w328) -> ()  [unwired: 1 in, 1 out]
                  }
                }
              }
            }
            n207 = Enqueue Element(queue=w299, element=w297, timeout in ms (-1)=1000 ("超时毫秒(-1)")) -> ()  [unwired: 1 in, 3 out]
          }
        }
      }
      frame "第二点校准失败" {
      }
      frame "放置第三点标液" {
        n208 = global read "多参数全局变量.vi" "多参数编号"() -> (w334:string)
        n209 = Format Into String(format string="编号：%s\n参数：%s\n信息：%s" ("格式字符串"), w334, "pH" ("输入 2"), "请把探头放入标液3中,放置好后按确认探头将继续校准,按取消探头将结束校准." ("消息")) -> (resulting string=w331:string)  [unwired: 2 in, 1 out]
        n210 = Two Button Dialog(message=w331) -> (T button?=w340:bool)  [unwired: 2 in]
        n211 = Select(t=校准步骤."第三点校准启动" ("元素"), s=w340, f=校准步骤."待机" ("元素")) -> (s? t:f=w337:T2)
        n212 = Enqueue Element(queue=w342, element=w337, timeout in ms (-1)=1000 ("超时毫秒(-1)")) -> ()  [unwired: 1 in, 3 out]
      }
      frame "第三点校准启动" {
        n213 = Greater Or Equal?(x=w352, y=60) -> (x >= y?=w353:bool)
        n214 = local read "最大值"() -> (w349:sgl)
        n215 = local read "最小值"() -> (w350:sgl)
        n216 = case shown="真" w353 {
          tunnel: [_ TRUE] -> w351
          frame False {
          }
          frame True {
          }
        }
        n217 = Subtract(x=w349, y=w350) -> (x-y=w348:sgl)
        n218 = Increment(x=w352) -> (x+1=w344:i32)
        n219 = Less Or Equal?(x=w348, y=10.0) -> (x <= y?=w356:bool)
        n220 = And(x=w356, y=w351) -> (x .and. y?=w347:bool)
        n221 = Greater Or Equal?(x=w344, y=180) -> (x >= y?=w345:bool)
        n222 = case shown="假" w347 {
          tunnel: w346 -> [w362 w374]
          tunnel: w345 -> [w363 _]
          tunnel: w344 -> [w361 _]
          tunnel: [w360 _] -> w343
          frame False {
            n223 = case shown="真" w363 {
              tunnel: w362 -> [_ w371]
              tunnel: w361 -> [w364 _]
              tunnel: [w364 _] -> w360
              frame False {
              }
              frame True {
                n224 = Enqueue Element(queue=w371, element=校准步骤."待机" ("元素")) -> ()  [unwired: 2 in, 3 out]
                n225 = global read "多参数全局变量.vi" "多参数编号"() -> (w366:string)
                n226 = Format Into String(format string="编号：%s\n参数：%s\n信息：%s" ("格式字符串"), w366, "pH" ("输入 2"), "第三点校准超时，请重新校准！" ("error source (\" \")")) -> (resulting string=w368:string)  [unwired: 2 in, 1 out]
                n227 = One Button Dialog(message=w368) -> ()  [unwired: 1 in, 1 out]
              }
            }
          }
          frame True {
            n228 = Enqueue Element(queue=w374, element=校准步骤."第三点校准写入" ("元素"), timeout in ms (-1)=1000 ("超时毫秒(-1)")) -> ()  [unwired: 1 in, 3 out]
          }
        }
        n229 = Format Into String(format string="正在进行第三点校准,校准可能需要几分钟,请耐性等待,已进行%d秒." ("格式字符串"), w343) -> (resulting string=w358:string)  [unwired: 2 in, 1 out]
      }
      frame "第三点校准写入" {
        n230 = Increment(x=w378) -> (x+1=w377:i32)
        n231 = case shown="1" w377 {
          tunnel: w376 -> [_ _ w387]
          frame 0, Default {
          }
          frame 1 {
            n232 = local read "当前信号值"() -> (→"第三点校准值":dbl)
          }
          frame 2 {
            n233 = local read "三点标液3"() -> (w382:u16)
            n234 = case shown="0, 默认" w382 {
              tunnel: [u16 49 ("数值") u16 50 ("数值") u16 51 ("数值") u16 52 ("数值") u16 53 ("数值") u16 54 ("数值") u16 55 ("数值") u16 56 ("数值")] -> w381
              frame 0, Default {
              }
              frame 1 {
              }
              frame 2 {
              }
              frame 3 {
              }
              frame 4 {
              }
              frame 5 {
              }
              frame 6 {
              }
              frame 7 {
              }
            }
            n235 = global read "多参数全局变量.vi" "MB session in"() -> (w384:refnum<class "MB_Master.lvclass">)
            n236 = call "0035H_pH_第三点校正指令写入.vi"("数值"=w381, "MB session in"=w384) -> ("error out"=w383:errorcluster)  [unwired: 8 in, 1 out]
            n237 = case shown="无错误" w383 {
              tunnel: [校准步骤."校准结果写入" ("元素") 校准步骤."第三点校准写入" ("元素")] -> w385
              frame No Error {
              }
              frame Error {
                n238 = global read "多参数全局变量.vi" "多参数编号"() -> (w398:string)
                n239 = Format Into String(format string="编号：%s\n参数：%s\n信息：%s" ("格式字符串"), w398, "pH" ("输入 2"), "第三点校准异常，请重新校准！" ("error source (\" \")")) -> (resulting string=w400:string)  [unwired: 2 in, 1 out]
                n240 = One Button Dialog(message=w400) -> ()  [unwired: 1 in, 1 out]
              }
            }
            n241 = Enqueue Element(queue=w387, element=w385, timeout in ms (-1)=1000 ("超时毫秒(-1)")) -> ()  [unwired: 1 in, 3 out]
          }
        }
      }
      frame "第三点校准失败" {
      }
      frame "校准结果写入" {
        n242 = call "时间延迟"() -> ("error out"=w404:errorcluster)  [unwired: 11 in]
        n243 = local read "校准模式"() -> (w411:enum16{"两点校准", "单点校准", "三点校准"})
        n244 = Enqueue Element(queue=w413, element=校准步骤."校准结束" ("元素")) -> ()  [unwired: 2 in, 3 out]
        n245 = case shown="\"单点校准\"" w411 {
          tunnel: [w416 w443] -> w405
          tunnel: w404 -> [_ _]
          frame "两点校准", Default {
            n246 = global read "国弘过程全局变量.vi" "pH"() -> (w415:T3)
            n247 = Unbundle By Name(w415) -> ("电极状态标志"=w414:u16)
            n248 = case shown="5" w414 {
              selector: w414 -> [w418 _ w429 _]
              tunnel: [w417 w425 w428 w438] -> w416
              frame 0, Default {
                n249 = case shown="1" w418 {
                  tunnel: ["校正未正常启动，请重新校正" "第一点校准通过" "第二点校准通过"] -> w417
                  frame 0, Default {
                  }
                  frame 1 {
                  }
                  frame 2 {
                  }
                }
              }
              frame 2 {
                n250 = local read "第一点校准值"() -> (w426:dbl)
                n251 = local read "第二点校准值"() -> (w423:dbl)
                n252 = local read "标液1"() -> (w427:dbl)
                n253 = local read "标液2"() -> (w422:dbl)
                n254 = Format Into String(format string="校准结果：第一点校准值=%f mV，第一点标准值=%f,第二点校准值=%f mV，第二点标准值=%f." ("提示"), w426, w427, w423, w422) -> (resulting string=w425:string)  [unwired: 2 in, 1 out]
              }
              frame 3, 4 {
                n255 = case shown="4" w429 {
                  tunnel: ["校正失败，电极零点超出范围" "校正失败，电极斜率超出范围"] -> w428
                  frame 3, Default {
                  }
                  frame 4 {
                  }
                }
              }
              frame 5 {
                n256 = local read "第一点校准值"() -> (w439:dbl)
                n257 = local read "第二点校准值"() -> (w437:dbl)
                n258 = local read "第三点校准值"() -> (w435:dbl)
                n259 = property on="三点标液1" class="Ring (严格)"() -> ("RingText.Text"=w434:string)  [unwired: 2 in, 2 out]
                n260 = property on="三点标液2" class="Ring (严格)"() -> ("RingText.Text"=w432:string)  [unwired: 2 in, 2 out]
                n261 = property on="三点标液3" class="Ring (严格)"() -> ("RingText.Text"=w433:string)  [unwired: 2 in, 2 out]
                n262 = Format Into String(format string="校准结果：第一点校准值=%f mV，第一点标准值=%s,第二点校准值=%f mV，第二点标准值=%s,第三点校准值=%f mV，第三点标准值=%s." ("提示"), w439, w434, w437, w432, w435, w433) -> (resulting string=w438:string)  [unwired: 2 in, 1 out]
              }
            }
          }
          frame "单点校准" {
            n263 = local read "第一点校准值"() -> (w442:dbl)
            n264 = local read "标液1"() -> (w440:dbl)
            n265 = Format Into String(format string="校准结果：校准值=%f，标准值=%f。" ("提示"), w442, w440) -> (resulting string=w443:string)  [unwired: 2 in, 1 out]
          }
        }
        n266 = global read "多参数全局变量.vi" "多参数编号"() -> (w408:string)
        n267 = Format Into String(format string="编号：%s\n参数：%s\n信息：%s" ("格式字符串"), w408, "pH" ("输入 2"), w405) -> (resulting string=w406:string)  [unwired: 2 in, 1 out]
        n268 = call "操作日志.vi"("table"="校准记录", "日志信息"=w406) -> ("error out"=w410:errorcluster)  [unwired: 9 in]
      }
      frame "校准结束" {
        n269 = local read "提示"() -> (w444:string)
      }
    }
    "提示" <- w124
  }
